vi "get_active_modes.vi"(8 "error in (no error)":errorcluster, 10 "active steps":u16, 11 "VISA Refnum in":refnum<visa-resource-name>) -> (0 "error out":errorcluster, 1 "modes":string[](array[string]), 2 "steps":u16[](array[numeric]), 3 "VISA Refnum out":refnum<visa-resource-name>)   [LabVIEW 2015]
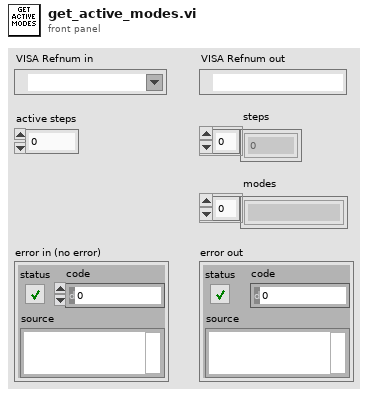
[diagram p1: front panel]
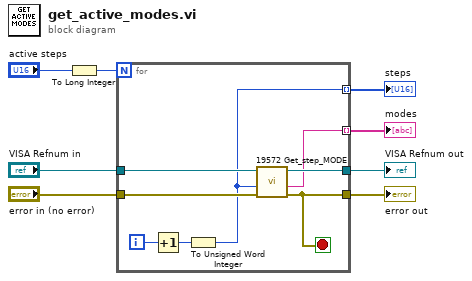
[diagram p0: block diagram]
diagram:
  n1 = To Long Integer(number="active steps") -> (32bit integer=w6:i32)
  n2 = for {
    N: w6 -> [_]
    tunnel: "VISA Refnum in" -> [w16]
    tunnel: "error in (no error)" -> [w15]
    tunnel: [w10] -> w4 mode=indexing
    tunnel: [w12] -> w3 mode=indexing
    tunnel: [w9] -> w5
    tunnel: [w11] -> w8
    i -> [w14]
    stop <- w9 stop-if-true
    n3 = Increment(x=w14) -> (x+1=w13:i32)
    n4 = To Unsigned Word Integer(number=w13) -> (unsigned 16bit integer=w12:u16)
    n5 = call "19572 Get_step_MODE.vi"("error in (no error)"=w15, "Step"=w12, "VISA resource in"=w16) -> ("error out"=w9:errorcluster, "Mode"=w10:string, "VISA resource out"=w11:refnum<visa-resource-name>)  [unwired: 6 in]
  }
  "VISA Refnum out" <- w8
  "error out" <- w5
  "modes" <- w4
  "steps" <- w3
